vi "fpga_is_finished.vi"(8 "error in":errorcluster, 11 "FPGA VI Reference in":T1) -> (0 "error out":errorcluster, 2 "Finished?":bool, 3 "FPGA VI Reference out":T1)   [LabVIEW 2011, in "Fiberscope_library.lvlib"]
uses:
  Fiberscope_library.lvlib
  typedefs/fpga_main_spiral_fpga_ref.ctl
  <vilib>/Utility/error.llb/Error Cluster From Error Code.vi
  <vilib>/rvi/errors/niLvFpgaAdjustHostInterfaceError.vi
  <vilib>/rvi/interface/nirviReadWriteControl/nirviReadWriteControl.xnode
  FPGA Bitfiles/FiberscopeRK1107_FPGATarget_fpgamainspiral_0DF2A7CB.lvbitx
  NiFpgaLv.dll
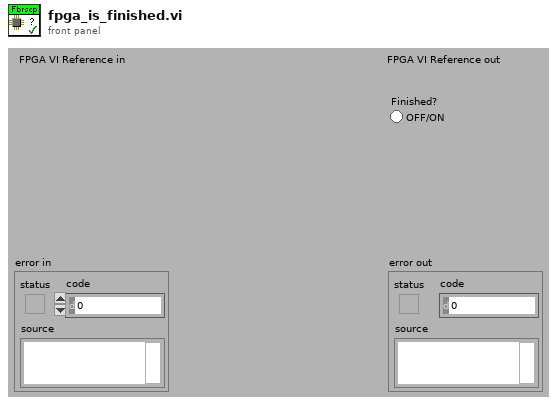
[diagram p1: front panel]
types:
  T1 = typedef "Fiberscope_library.lvlib/fpga_main_spiral_fpga_ref.ctl" = refnum<k20>
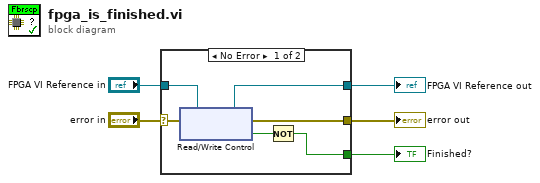
[diagram p0: block diagram]
diagram:
  n1 = case shown="No Error" "error in" {
    selector: "error in" -> [w9 w13]
    tunnel: [w10 w13] -> w4
    tunnel: "FPGA VI Reference in" -> [w8 w12]
    tunnel: [w11 w12] -> w2
    tunnel: [w7 _] -> w1
    frame No Error {
      n2 = xnode "Read/Write Control"("FPGA VI Reference In"=w8, "error in"=w9) -> ("FPGA VI Reference Out"=w11:T1, "error out"=w10:errorcluster, "Scanning?"=w6:bool)
      n3 = Not(x=w6) -> (.not. x?=w7:bool)
    }
    frame Error {
    }
  }
  "error out" <- w4
  "FPGA VI Reference out" <- w2
  "Finished?" <- w1
